vi "Clear.vi"(8 "error in (no error)":errorcluster, 11 "reference in":refnum<class "Console.lvclass">) -> (0 "error out":errorcluster, 3 "reference out":refnum<class "Console.lvclass">)   [LabVIEW 2018, in "Console.lvclass"]
doc: "Clear the console of all lines"
uses:
  Console.lvclass
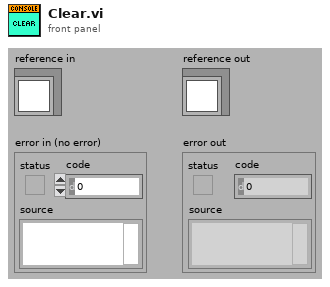
[diagram p1: front panel]
types:
  T1 = typedef "Console.lvclass/ObjectAttributes.ctl" = cluster{"data":string, "count":dbl}
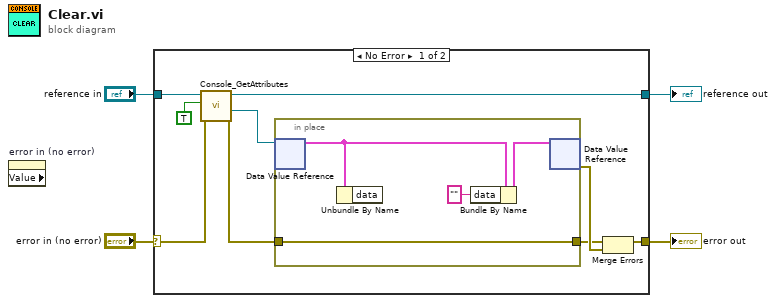
[diagram p0: block diagram]
diagram:
  n1 = property on="error in (no error)" class="Clust (strict)" props=["Value"]() -> ()  [unwired: 2 in, 3 out]
  n2 = case shown="No Error" "error in (no error)" {
    selector: "error in (no error)" -> [w8 w19]
    tunnel: [w12 w19] -> w3
    tunnel: [w10 w18] -> w1
    tunnel: "reference in" -> [w11 w18]
    frame No Error {
      n3 = call "Console_GetAttributes.vi"("error in (no error)"=w8, "OnlyGetDvrReference(False)"=TRUE, "reference in"=w11) -> ("error out"=w7:errorcluster, "DataRef"=w9:refnum<data-value>, "reference out"=w10:refnum<class "Console.lvclass">)  [unwired: 5 in, 1 out]
      n4 = in-place {
        in-place-border: w7 -> [w16]
        in-place-border: [w16] -> w6
        n5 = in-place-dvr #1(w9) -> (w15:T1)  [unwired: 1 out]
        n6 = Unbundle By Name(w15) -> ()  [unwired: 1 out]
        n7 = Bundle By Name(cluster=w15, "data"="") -> (w17:T1)
        n8 = in-place-dvr #1(w17) -> (w13:errorcluster)  [unwired: 1 out]
      }
      n9 = Merge Errors(w6, w13) -> (w12:errorcluster)
    }
    frame Error {
    }
  }
  "error out" <- w3
  "reference out" <- w1
